vi "ProdaNG.ProcessStep.Get.vi"(8 "error in (no error)":errorcluster, 10 "processStepId":i32, 11 "dbHandleIn":i32) -> (0 "error out":errorcluster, 2 "ProcessStep":T1, 3 "dbHandle":i32)   [LabVIEW 2016]
doc: "This function returns a product structure for a product, which is identified by a part and a serial number.\nImportant information: The field 'individual' was taken over from the field 'allgemein' of the legacy data directly. Because of this most products have the value 0 further on and only a few the value 1. \nParameter:\nhandle is an Integer, which is returned by the function Login() at the creation of a new connection.\nwabcoPartId is the Id of the part.\nserialNumber is the serial number of the product for the part above.\nproduct is a pointer on a product structure, which is filled if the returncode is 0. The structure must be defined in the calling program.\n\nReturncodes:\n0 No error\n< 0 ORACLE Error code\n6 (ERROR_INVALID_HANDLE) in case of an invalid handle\n1403 Record does not exist"
uses:
  Controls/ProdaNG.ProcessStep.ctl
  Controls/ProdaNG.ProcessStepSize.ctl
  prodllNG.dll
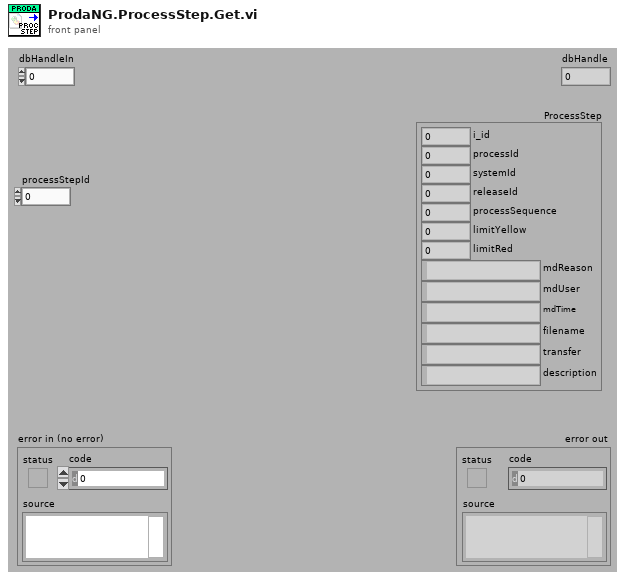
[diagram p1: front panel]
types:
  T1 = typedef "ProdaNG.ProcessStep.ctl" = cluster{"i_id":i32, "processId":i32, "systemId":i32, "releaseId":i32, "processSequence":i32, "limitYellow":dbl, "limitRed":dbl, "mdReason":string, "mdUser":string, "mdTime":string, "filename":string, "transfer":string, "description":string}
  T2 = typedef "ProdaNG.ProcessStepSize.ctl" = cluster{"i_id":i32, "processId":i32, "systemId":i32, "releaseId":i32, "processSequence":i32, "limitYellow":i32, "limitRed":i32, "mdReason":i32, "mdUser":i32, "mdTime":i32, "filename":i32, "transfer":i32, "description":i32}
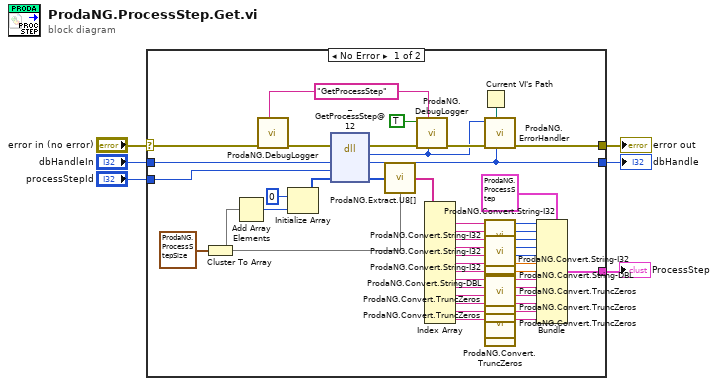
[diagram p0: block diagram]
diagram:
  n1 = case shown="No Error" "error in (no error)" {
    selector: "error in (no error)" -> [w48 w55]
    tunnel: [w53 w55] -> w5
    tunnel: "dbHandleIn" -> [w50 w54]
    tunnel: [w51 w54] -> w3
    tunnel: "processStepId" -> [w42 _]
    tunnel: [w9 _] -> w1
    frame No Error {
      w44 = "GetProcessStep" ("cmd")
      n2 = Cluster To Array(cluster=T2 {"i_id"=4, "processId"=4, "systemId"=4, "releaseId"=4, "processSequence"=4, "limitYellow"=8, "limitRed"=8, "mdReason"=514, "mdUser"=22, "mdTime"=24, "filename"=258, "transfer"=2, "description"=514} ("ProcStepSize")) -> (array=w11:i32[])
      n3 = Add Array Elements(numeric array=w11) -> (sum=w12:i32)
      n4 = call "ProdaNG.DebugLogger.vi"("cmd"=w44, "error in (no error)"=w48) -> ("error out"=w47:errorcluster)  [unwired: 9 in]
      n5 = Initialize Array(u8 0 ("element"), w12) -> (w10:u8[])
      n6 = dll-call lib="D:/svn/LineTraceSystem/SOFTWARE/sources/Database/ProdaNG/prodllNG.dll" fn="_GetProcessStep@12" ("ProDLL wrapper.dll:ProDLL_wrapper_GetWabcoParts_GetData")(error in=w47, "dbHandle"=w50, "processStepId"=w42, "processStep"=w10) -> (error out=w46:errorcluster, "return type"=w43:i32, "dbHandle"=w51:i32, "processStep"=w8:u8[])  [unwired: 3 in, 1 out]
      n7 = call "ProdaNG.Extract.U8[].vi"("unsigned byte array"=w8, "Sizes"=w11) -> ("Elements"=w7:string[])
      n8 = call "ProdaNG.DebugLogger.vi"("return type"=w43, "cmd"=w44, "error in (no error)"=w46, "done? (F)"=TRUE) -> ("error out"=w45:errorcluster)  [unwired: 7 in]
      n9 = Index Array(array=w7) -> (element #1=w30:string, element #2=w29:string, element #3=w39:string, element #4=w36:string, element #5=w33:string, element #6=w35:string, element #7=w28:string, element #8=w27:string, element #9=w24:string, element #10=w22:string, element #11=w20:string, element #12=w18:string, element #13=w16:string)  [unwired: 13 in]
      n10 = Current VI's Path() -> (path=w52:path)
      n11 = call "ProdaNG.ErrorHandler.vi"("dbHandleIn"=w51, "Path"=w52, "error in"=w45, "output_parameter"=w43) -> ("error out"=w53:errorcluster)  [unwired: 7 in]
      n12 = call "ProdaNG.Convert.String-I32.vi"("unsigned byte string"=w30) -> ("32bit integer"=w32:i32)  [unwired: 10 in]
      n13 = call "ProdaNG.Convert.String-I32.vi"("unsigned byte string"=w29) -> ("32bit integer"=w31:i32)  [unwired: 10 in]
      n14 = call "ProdaNG.Convert.String-I32.vi"("unsigned byte string"=w39) -> ("32bit integer"=w38:i32)  [unwired: 10 in]
      n15 = call "ProdaNG.Convert.String-I32.vi"("unsigned byte string"=w36) -> ("32bit integer"=w37:i32)  [unwired: 10 in]
      n16 = call "ProdaNG.Convert.String-I32.vi"("unsigned byte string"=w33) -> ("32bit integer"=w14:i32)  [unwired: 10 in]
      n17 = call "ProdaNG.Convert.String-DBL.vi"("unsigned byte string"=w35) -> ("dbl integer"=w34:dbl)  [unwired: 10 in]
      n18 = call "ProdaNG.Convert.String-DBL.vi"("unsigned byte string"=w28) -> ("dbl integer"=w26:dbl)  [unwired: 10 in]
      n19 = call "ProdaNG.Convert.TruncZeros.vi"("string with \\0s"=w27) -> ("LV string"=w25:string)  [unwired: 10 in]
      n20 = call "ProdaNG.Convert.TruncZeros.vi"("string with \\0s"=w24) -> ("LV string"=w23:string)  [unwired: 10 in]
      n21 = call "ProdaNG.Convert.TruncZeros.vi"("string with \\0s"=w22) -> ("LV string"=w21:string)  [unwired: 10 in]
      n22 = call "ProdaNG.Convert.TruncZeros.vi"("string with \\0s"=w20) -> ("LV string"=w19:string)  [unwired: 10 in]
      n23 = call "ProdaNG.Convert.TruncZeros.vi"("string with \\0s"=w18) -> ("LV string"=w17:string)  [unwired: 10 in]
      n24 = call "ProdaNG.Convert.TruncZeros.vi"("string with \\0s"=w16) -> ("LV string"=w15:string)  [unwired: 10 in]
      n25 = Bundle(cluster=T1 {"i_id"=0, "processId"=0, "systemId"=0, "releaseId"=0, "processSequence"=0, "limitYellow"=0.0, "limitRed"=0.0, "mdReason"="", "mdUser"="", "mdTime"="", "filename"="", "transfer"="", "description"=""} ("ProcessStep"), "i_id"=w32, "processId"=w31, "systemId"=w38, "releaseId"=w37, "processSequence"=w14, "limitYellow"=w34, "limitRed"=w26, "mdReason"=w25, "mdUser"=w23, "mdTime"=w21, "filename"=w19, "transfer"=w17, "description"=w15) -> (w9:T1)
    }
    frame Error {
    }
  }
  "error out" <- w5
  "dbHandle" <- w3
  "ProcessStep" <- w1
